vi "Set Configuration Parameter - Integer.vi"(7 "Section":string, 8 "error in (no error)":errorcluster, 9 "Value":i32, 10 "Key":string, 11 "Ethernet in":refnum<class "ENET_BS1201.lvclass">) -> (0 "error out":errorcluster, 3 "Ethernet out":refnum<class "ENET_BS1201.lvclass">)   [LabVIEW 2021, in "BS120x Driver.lvlib" / "ENET_BS1201.lvclass"]
uses:
  ENET_BS1201.lvclass
  C:/Users/Public/Documents/Projects/7100-00109 SW BS1201 LV Driver/trunk/source/ENET_BS120x/ENET_BS120x.lvclass
  ENET_BS1201.lvclass/ENET_BS1201.ctl
  ENET_BS120x/ENET_BS120x.lvclass
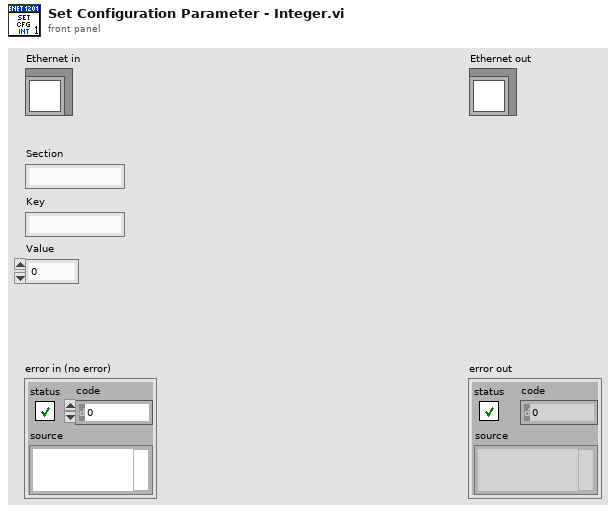
[diagram p1: front panel]
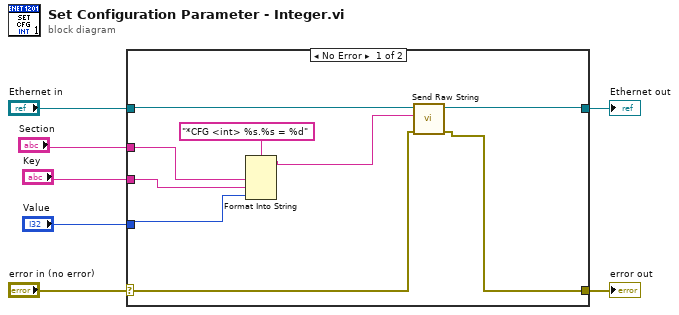
[diagram p0: block diagram]
diagram:
  n1 = case shown="No Error" "error in (no error)" {
    selector: "error in (no error)" -> [w9 w18]
    tunnel: [w8 w18] -> w6
    tunnel: [w15 w17] -> w4
    tunnel: "Ethernet in" -> [w16 w17]
    tunnel: "Section" -> [w13 _]
    tunnel: "Key" -> [w12 _]
    tunnel: "Value" -> [w10 _]
    frame No Error {
      n2 = Format Into String(format string="*CFG <int> %s.%s = %d", w13, w12, w10) -> (resulting string=w11:string)  [unwired: 2 in, 1 out]
      n3 = call "Send Raw String.vi"("error in (no error)"=w9, "String Data"=w11, "ENET in"=w16) -> ("error out"=w8:errorcluster, "ENET out"=w15:refnum<class "ENET_BS1201.lvclass">)  [unwired: 7 in]
    }
    frame Error {
    }
  }
  "error out" <- w6
  "Ethernet out" <- w4
